vi "Memory.Pointer.Write.Safe.1D.U32.vi"(8 "error in (no error)":errorcluster, 9 "count":u64 format="%d elements", 10 "buffer in":u32[](array[numeric]), 11 "pointer in":refnum<class "Memory.Pointer.lvclass">) -> (0 "error out":errorcluster, 2 "buffer out":u32[](array[numeric]), 3 "pointer out":refnum<class "Memory.Pointer.lvclass">)   [LabVIEW 2016, in "Memory Manager.lvlib" / "Memory.Pointer.lvclass"]
doc: "Writes <b>count</b> elements from the provided <b>buffer</b> to the address specified by <b>pointer</b>.\n\n<b>Note:</b> This VI is <b>safe</b>.\n\nSafe means that this function evaluates the size parameter of <b>pointer</b> to ensure that is inbounds of allocated memory before peforming a memory read/write. Reading/writing more data to a pointer than it has allocated can corrupt or crash LabVIEW."
uses:
  Memory.Pointer.lvclass
  Memory.Pointer.lvclass/Memory.Pointer.ctl
  Accessors/Get Address.vi
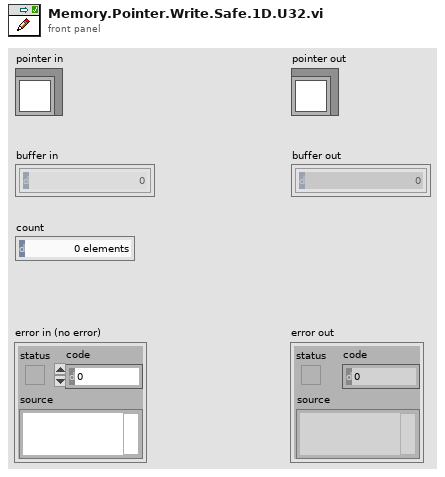
[diagram p1: front panel]
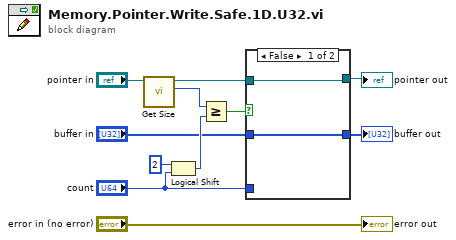
[diagram p0: block diagram]
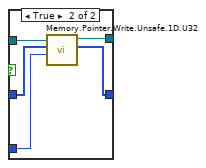
[diagram p2: hidden frame]
diagram:
  n1 = call "Get Size.vi"("Pointer in"="pointer in") -> ("size"=w9:u64, "Pointer out"=w6:refnum<class "Memory.Pointer.lvclass">)  [unwired: 8 in, 1 out]
  n2 = Logical Shift(y=i16 2, x="count") -> (x << y=w8:u64)
  n3 = Greater Or Equal?(x=w9, y=w8) -> (x >= y?=w7:bool)
  n4 = case shown="False" w7 {
    tunnel: w6 -> [w13 w18]
    tunnel: "buffer in" -> [w12 w17]
    tunnel: "count" -> [_ w16]
    tunnel: [w12 w15] -> w3
    tunnel: [w13 w14] -> w2
    frame False {
    }
    frame True {
      n5 = call "Memory.Pointer.Write.Unsafe.1D.U32.vi"("count"=w16, "buffer in"=w17, "pointer in"=w18) -> ("buffer out"=w15:u32[], "pointer out"=w14:refnum<class "Memory.Pointer.lvclass">)  [unwired: 6 in, 1 out]
    }
  }
  "pointer out" <- w2
  "buffer out" <- w3
  "error out" <- "error in (no error)"
